vi "Save_full_Res_rows.vi"(2 "Selected Rows":i32[](array[numeric]), 3 "Filename to write":path, 4 "Filename Orig":path) -> ()   [LabVIEW 2020]
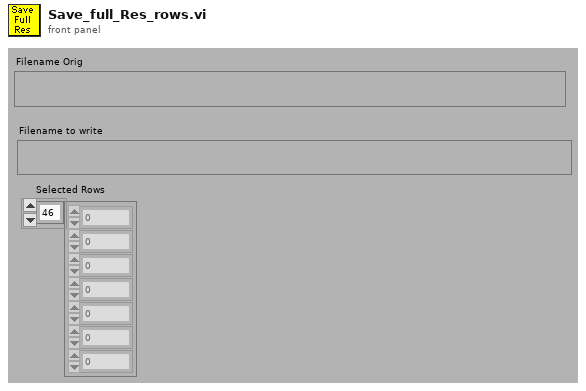
[diagram p1: front panel]
types:
  T1 = enum16{"read/write", "read-only", "write-only", "write-only (truncate)"}
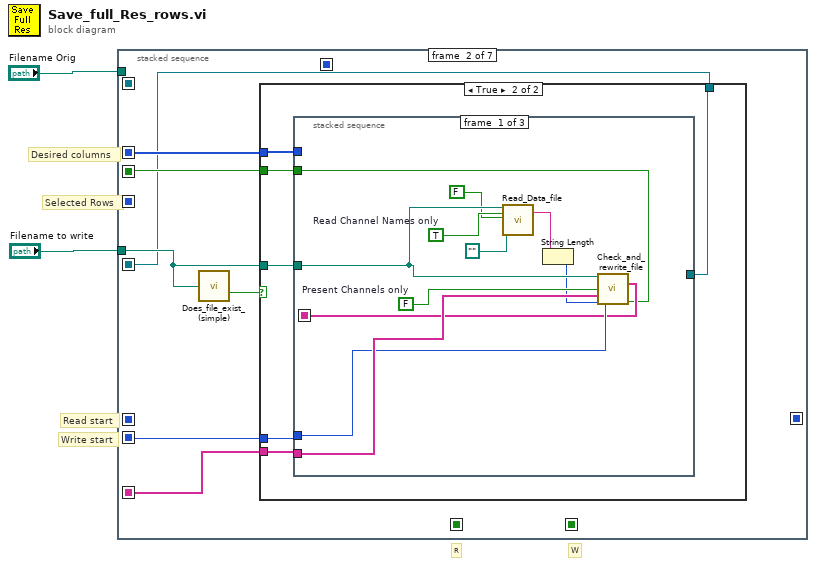
[diagram p0: block diagram]
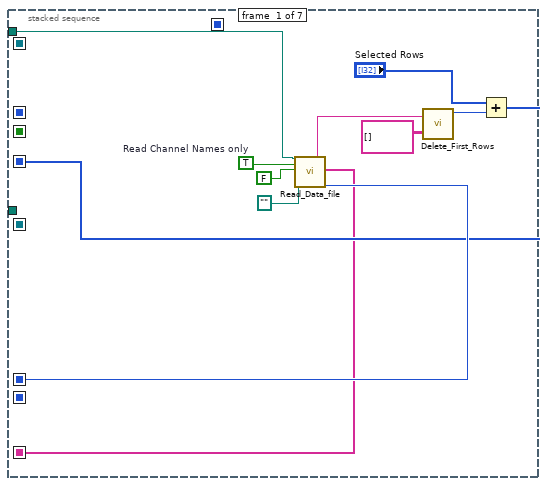
[diagram p2: hidden frame]
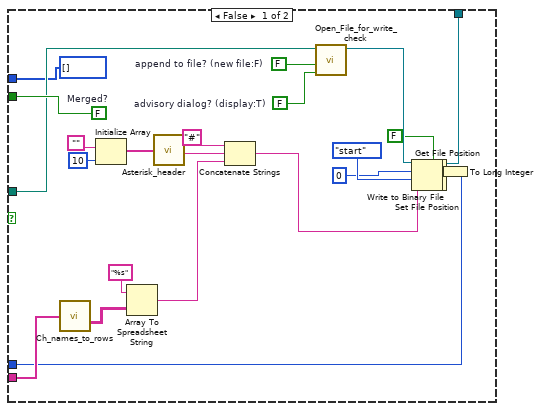
[diagram p3: hidden frame]
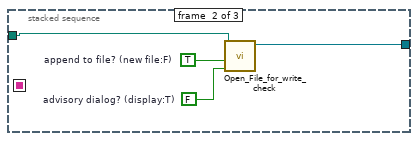
[diagram p4: hidden frame]
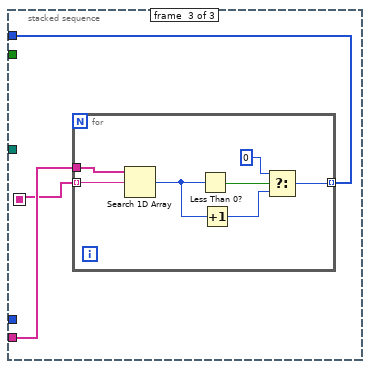
[diagram p5: hidden frame]
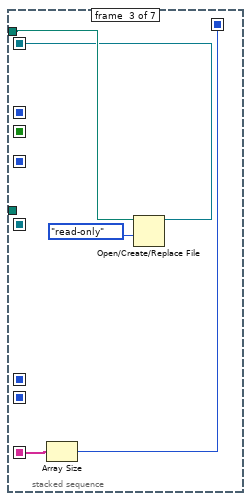
[diagram p6: hidden frame]
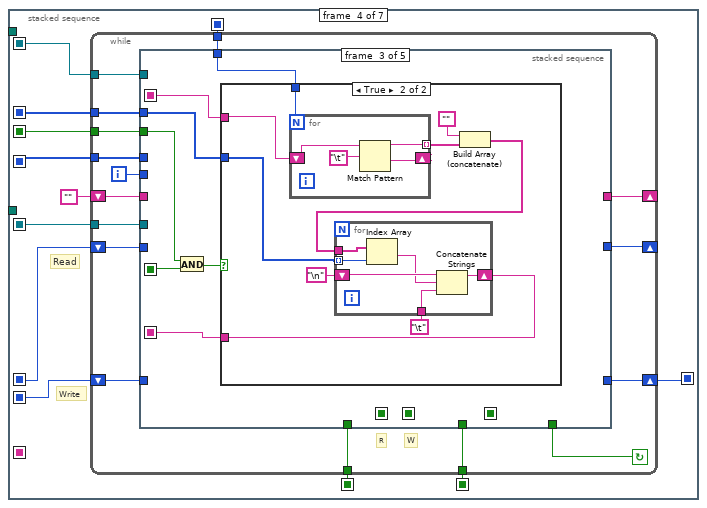
[diagram p7: hidden frame]
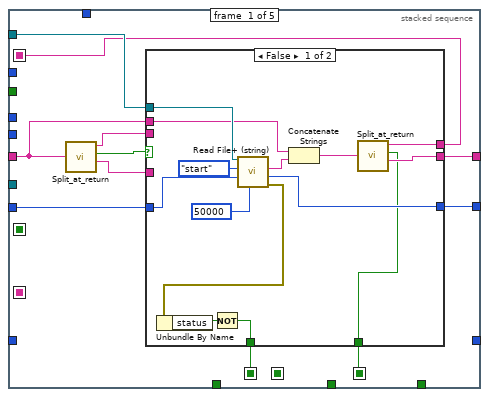
[diagram p8: hidden frame]
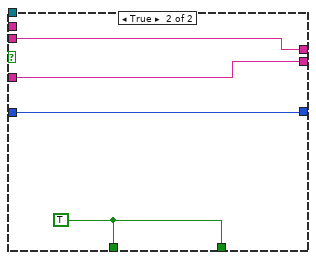
[diagram p9: hidden frame]
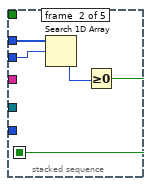
[diagram p10: hidden frame]
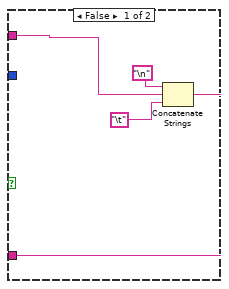
[diagram p11: hidden frame]
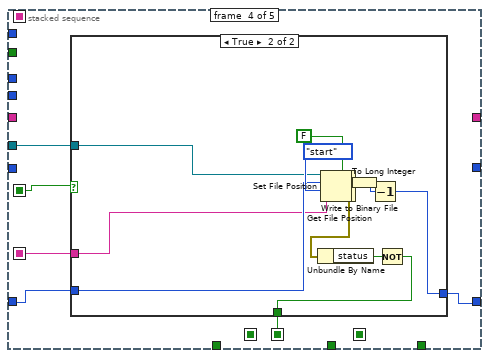
[diagram p12: hidden frame]
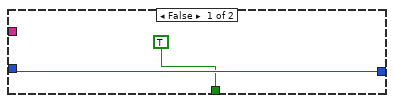
[diagram p13: hidden frame]
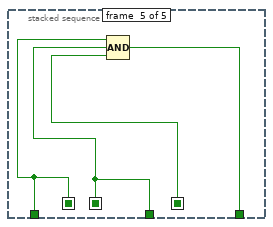
[diagram p14: hidden frame]
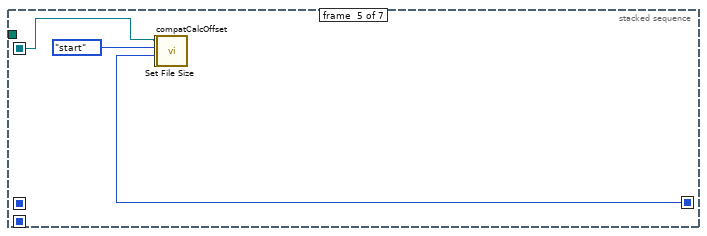
[diagram p15: hidden frame]
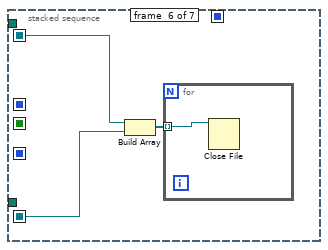
[diagram p16: hidden frame]
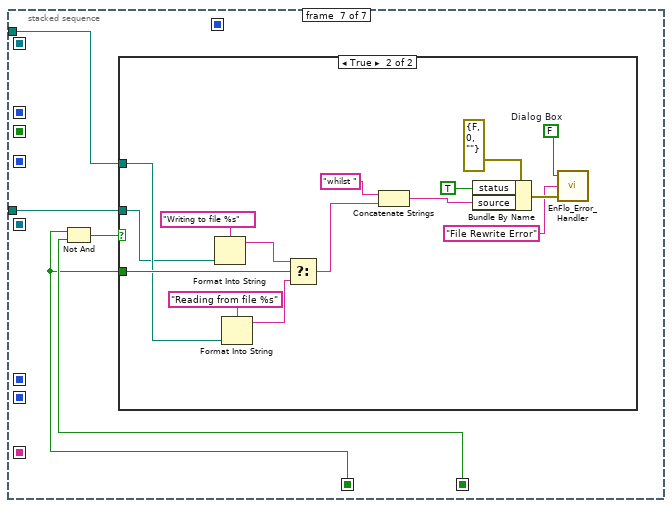
[diagram p17: hidden frame]
diagram:
  # "Desired columns"
  # "Selected Rows"
  # "Read start"
  # "Write start"
  # "W"
  # "R"
  n1 = stacked-sequence {
    seq-local: [_ _ w80 _ _ _ _] -> [_ _ _ w86 _ w209 _]
    seq-local: [w10 _ _ _ _ _ _] -> [_ _ _ w89 _ _ _]
    seq-local: [_ _ _ w93 _ _ _] -> [_ _ _ _ _ _ w213]
    seq-local: [_ _ _ w92 _ _ _] -> [_ _ _ _ _ _ w215]
    seq-local: [_ _ _ w91 _ _ _] -> [_ _ _ _ w206 _ _]
    seq-local: [w5 _ _ _ _ _ _] -> [_ _ _ w90 _ _ _]
    seq-local: [_ w16 _ _ _ _ _] -> [_ _ _ w88 _ _ _]
    seq-local: [w4 _ _ _ _ _ _] -> [_ w19 w79 _ _ _ _]
    seq-local: [_ w18 _ _ _ _ _] -> [_ _ _ w83 _ _ _]
    seq-local: [_ w17 _ _ _ _ _] -> [_ _ _ w84 _ _ _]
    seq-local: [_ w14 _ _ _ _ _] -> [_ _ _ w87 w204 w207 _]
    seq-local: [_ _ w78 _ _ _ _] -> [_ _ _ w85 _ _ _]
    tunnel: "Filename Orig" -> [w11 _ w81 _ _ _ w212]
    tunnel: "Filename to write" -> [_ w15 _ _ _ _ w211]
    frame #0 {
      w12 = TRUE  # Read Channel Names only
      n2 = call "Read_Data_file.vi"("Results file"=w11, "Read Channel Names only"=w12, "Delete First Rows?"=FALSE, "Template File"=path "") -> ("Filetype"=w9:string, "Ch names Out"=w4:string[], "mark after read (chars.)"=w10:i32)  [unwired: 3 in, 10 out]
      n3 = call "Delete_First_Rows.vi"("File Type (Default: AutoTrim)"=w9, "Data In"=string[][] []) -> ("Rows removed"=w8:i32)  [unwired: 2 out]
      n4 = Add(x="Selected Rows", y=w8) -> (x+y=w5:i32[])
    }
    frame #1 {
      n5 = call "Does_file_exist_(simple).vi"("Pathname"=w15) -> ("exists?"=w20:bool)
      n6 = case shown="True" w20 {
        tunnel: w15 -> [w34 w52]
        tunnel: w19 -> [w45 w51]
        tunnel: [i32[] [] w48] -> w18
        tunnel: [w46 w47] -> w17
        tunnel: [w28 w50] -> w16
        tunnel: [w29 w49] -> w14
        frame False {
          w35 = FALSE  # advisory dialog? (display:T)
          w36 = FALSE  # append to file? (new file:F)
          w46 = FALSE  # Merged?
          n7 = call "Ch_names_to_rows.vi"("Channel Names"=w45) -> ("3 Row names"=w38:string[][])
          n8 = Initialize Array("", 10 ("Dimension Size")) -> (w42:string[])
          n9 = Array To Spreadsheet String(array=w38, 3:"%s" ("format string")) -> (spreadsheet string=w37:string)  [unwired: 1 out]
          n10 = call "Asterisk_header.vi"("Channel names"=w42) -> ("Header string"=w41:string)
          n11 = Concatenate Strings("#" ("Substring"), w41, w37) -> (w30:string)
          n12 = call "Open_File_for_write_check.vi"("advisory dialog? (display:T)"=w35, "append to file? (new file:F)"=w36, "file path"=w34) -> ("refnum"=w31:refnum<file>)  [unwired: 8 out]
          n13 = Set File Position(offset (in bytes) (0)=0 ("pos offset (0)"), refnum=w31, from (0:start)=enum16{"start", "end", "current"}."start" ("pos mode (0:2)")) -> (refnum out=w26:refnum<file>, error out=w25:errorcluster)  [unwired: 1 in]
          n14 = Write to Binary File(file (use dialog)=w26, data=w30, error in=w25, 5:FALSE ("prepend array or string size? (T)")) -> (refnum out=w24:refnum<file>, error out=w23:errorcluster)  [unwired: 3 out]
          n15 = Get File Position(4:w23, 7:w24) -> (2:w22:i64, 3:w29:refnum<file>)  [unwired: 1 out]
          n16 = To Long Integer(number=w22) -> (32bit integer=w28:i32)
        }
        frame True {
          n17 = stacked-sequence {
            seq-local: [w60 _ _] -> [_ _ w69]
            tunnel: w52 -> [w56 w65 _]
            tunnel: w51 -> [w62 _ w70]
            tunnel: [w61 _ _] -> w50
            tunnel: [_ w64 _] -> w49
            tunnel: [_ _ w68] -> w48
            tunnel: [w59 _ _] -> w47
            frame #0 {
              w58 = TRUE  # Read Channel Names only
              w63 = FALSE  # Present Channels only
              n18 = call "Read_Data_file.vi"("Results file"=w56, "Read Channel Names only"=w58, "Delete First Rows?"=FALSE, "Template File"=path "") -> ("String Before"=w55:string)  [unwired: 3 in, 12 out]
              n19 = String Length(string=w55) -> (length=w54:i32)
              n20 = call "Check_and_rewrite_file.vi"("Filename"=w56, "Present Channels only"=w63, "Present Channels"=w62, "Start of read offset (chars.: 0)"=w54) -> ("Merged Channels"=w60:string[], "Current file size (bytes)"=w61:i64, "Merged?"=w59:bool)  [unwired: 9 out]
            }
            frame #1 {
              w66 = FALSE  # advisory dialog? (display:T)
              w67 = TRUE  # append to file? (new file:F)
              n21 = call "Open_File_for_write_check.vi"("advisory dialog? (display:T)"=w66, "append to file? (new file:F)"=w67, "file path"=w65) -> ("refnum"=w64:refnum<file>)  [unwired: 8 out]
            }
            frame #2 {
              n22 = for {
                tunnel: w70 -> [w77]
                tunnel: w69 -> [w76] mode=indexing
                tunnel: [w71] -> w68 mode=indexing
                n23 = Search 1D Array(1D array=w77, element=w76) -> (index of element=w74:i32)  [unwired: 1 out]
                n24 = Less Than 0?(x=w74) -> (x < 0?=w75:bool)
                n25 = Increment(x=w74) -> (x+1=w73:i32)
                n26 = Select(t=0, s=w75, f=w73) -> (s? t:f=w71:i32)
              }
            }
          }
        }
      }
    }
    frame #2 {
      n27 = Array Size(array=w79) -> (size(s)=w78:i32)
      n28 = Open/Create/Replace File(file path (use dialog)=w81, access (0:read/write)=T1."read-only" ("open mode (0)")) -> (refnum out=w80:refnum<file>)  [unwired: 1 in, 5 out]
    }
    frame #3 {
      # "Write"
      # "Read"
      n29 = while {
        tunnel: [w101] -> w92
        tunnel: [w102] -> w93
        shift-left: w88 -> [w105]
        shift-right: [w104] -> w91
        tunnel: w86 -> [w107]
        shift-left: w89 -> [w109]
        shift-right: [w108] -> _
        shift-left: "" -> [w110]
        shift-right: [w106] -> _
        tunnel: w90 -> [w100]
        tunnel: w87 -> [w98]
        tunnel: w85 -> [w97]
        tunnel: w84 -> [w96]
        tunnel: w83 -> [w95]
        i -> [w99]
        stop <- w103 continue-if-true
        # "R"
        # "W"
        n30 = stacked-sequence {
          seq-local: [w113 _ _ _ _] -> [_ _ w144 _ _]
          seq-local: [_ _ _ w176 _] -> [_ _ _ _ w197]
          seq-local: [w114 _ _ _ _] -> [_ _ _ _ w199]
          seq-local: [w115 _ _ _ _] -> [_ _ _ _ w198]
          seq-local: [_ w140 _ _ _] -> [_ _ w148 w179 _]
          seq-local: [_ _ w149 _ _] -> [_ _ _ w175 _]
          tunnel: w110 -> [w118 _ _ _ _]
          tunnel: w109 -> [w121 _ _ _ _]
          tunnel: [w120 _ _ _ _] -> w108
          tunnel: w107 -> [w119 _ _ _ _]
          tunnel: [w117 _ _ _ _] -> w106
          tunnel: w105 -> [_ _ _ w178 _]
          tunnel: [_ _ _ w177 _] -> w104
          tunnel: [_ _ _ _ w200] -> w103
          tunnel: [_ _ _ _ w198] -> w102
          tunnel: [_ _ _ _ w197] -> w101
          tunnel: w100 -> [_ w143 _ _ _]
          tunnel: w99 -> [_ w142 _ _ _]
          tunnel: w98 -> [_ _ _ w174 _]
          tunnel: w97 -> [_ _ w150 _ _]
          tunnel: w96 -> [_ _ w147 _ _]
          tunnel: w95 -> [_ _ w145 _ _]
          frame #0 {
            n31 = call "Split_at_return.vi"("String"=w118) -> ("before substring"=w112:string, "Matched?"=w111:bool, "after substring"=w116:string)  [unwired: 1 in, 1 out]
            n32 = case shown="False" w111 {
              tunnel: w121 -> [w135 w139]
              tunnel: [w133 w139] -> w120
              tunnel: w119 -> [w132 _]
              tunnel: w118 -> [w130 _]
              tunnel: [w128 w138] -> w117
              tunnel: w116 -> [_ w138]
              tunnel: [w125 w137] -> w115
              tunnel: [w123 w137] -> w114
              tunnel: [w124 w136] -> w113
              tunnel: w112 -> [_ w136]
              frame False {
                n33 = call <vilib>:"Read File+ (string).vi"("count"=50000, "pos offset (bytes:0)"=w135, "pos mode (rel. to current:2)"=enum16{"start", "end", "current"}."start", "refnum"=w132) -> ("error out"=w127:errorcluster, "mark after read (bytes)"=w133:i32, "string"=w131:string)  [unwired: 1 in, 4 out]
                n34 = Unbundle By Name(w127) -> ("status"=w126:bool)
                n35 = Not(x=w126) -> (.not. x?=w125:bool)
                n36 = Concatenate Strings(w130, w131) -> (w129:string)
                n37 = call "Split_at_return.vi"("String"=w129) -> ("before substring"=w124:string, "Matched?"=w123:bool, "after substring"=w128:string)  [unwired: 1 in, 1 out]
              }
              frame True {
                w137 = TRUE
              }
            }
          }
          frame #1 {
            n38 = Search 1D Array(1D array=w143, element=w142) -> (index of element=w141:i32)  [unwired: 1 out]
            n39 = Greater Or Equal To 0?(x=w141) -> (x >= 0?=w140:bool)
          }
          frame #2 {
            n40 = And(x=w147, y=w148) -> (x .and. y?=w146:bool)
            n41 = case shown="True" w146 {
              tunnel: w144 -> [w153 w158]
              tunnel: w145 -> [_ w157]
              tunnel: w150 -> [_ w156]
              tunnel: [w152 w155] -> w149
              frame False {
                n42 = Concatenate Strings("\n", w153, "\t") -> (w152:string)
              }
              frame True {
                n43 = for {
                  N: w156 -> [_]
                  shift-right: [w165] -> _
                  shift-left: w158 -> [w166]
                  tunnel: [w164] -> w159 mode=indexing
                  n44 = Match Pattern(string=w166, regular expression="\t") -> (before substring=w164:string, after substring=w165:string)  [unwired: 3 out]
                }
                n45 = Build Array (concatenate)("", w159) -> (w163:string[])
                n46 = for {
                  tunnel: w157 -> [w173] mode=indexing
                  tunnel: w163 -> [w172]
                  shift-right: [w168] -> w155
                  shift-left: "\n" -> [w171]
                  tunnel: "\t" -> [w169]
                  n47 = Index Array(array=w172, index=w173) -> (element=w170:string)
                  n48 = Concatenate Strings(w171, w170, w169) -> (w168:string)
                }
              }
            }
          }
          frame #3 {
            n49 = case shown="True" w179 {
              tunnel: w178 -> [w181 w194]
              tunnel: [w181 w193] -> w177
              tunnel: [TRUE w190] -> w176
              tunnel: w175 -> [_ w189]
              tunnel: w174 -> [_ w188]
              frame False {
              }
              frame True {
                n50 = Set File Position(offset (in bytes) (0)=w194, refnum=w188, from (0:start)=enum16{"start", "end", "current"}."start" ("pos mode (0:2)")) -> (refnum out=w187:refnum<file>, error out=w186:errorcluster)  [unwired: 1 in]
                n51 = Write to Binary File(file (use dialog)=w187, data=w189, error in=w186, 5:FALSE ("prepend array or string size? (T)")) -> (refnum out=w185:refnum<file>, error out=w184:errorcluster)  [unwired: 3 out]
                n52 = Get File Position(4:w184, 7:w185) -> (0:w191:errorcluster, 2:w183:i64)  [unwired: 1 out]
                n53 = Unbundle By Name(w191) -> ("status"=w192:bool)
                n54 = To Long Integer(number=w183) -> (32bit integer=w196:i32)
                n55 = Decrement(x=w196) -> (x-1=w193:i32)
                n56 = Not(x=w192) -> (.not. x?=w190:bool)
              }
            }
          }
          frame #4 {
            n57 = Compound Arithmetic op=AND(w198, w197, w199) -> (w200:bool)
          }
        }
      }
    }
    frame #4 {
      n58 = call <vilib>:"compatCalcOffset.vi"("pos offset (0)"=w206, "pos mode (0:1)"=enum16{"start", "end", "current"}."start", "refnum"=w204) -> ("error out"=w203:errorcluster, "offset"=w202:i32, "dup refnum"=w201:refnum<file>)  [unwired: 1 in, 5 out]
      n59 = Set File Size(4:w203, 6:w202, 7:w201) -> ()  [unwired: 2 out]
    }
    frame #5 {
      n60 = Build Array(w209, w207) -> (w208:refnum<file>[])
      n61 = for {
        tunnel: w208 -> [w210] mode=indexing
        n62 = Close File(refnum=w210) -> ()  [unwired: 1 in, 2 out]
      }
    }
    frame #6 {
      n63 = Not And(1:w215, 2:w213) -> (0:w214:bool)
      n64 = case shown="True" w214 {
        tunnel: w213 -> [_ w230]
        tunnel: w212 -> [_ w220]
        tunnel: w211 -> [_ w217]
        frame False {
        }
        frame True {
          w225 = FALSE  # Dialog Box
          n65 = Format Into String(format string="Writing to file %s", w217) -> (resulting string=w216:string)  [unwired: 2 in, 1 out]
          n66 = Format Into String(format string="Reading from file %s", w220) -> (resulting string=w219:string)  [unwired: 2 in, 1 out]
          n67 = Select(t=w216, s=w230, f=w219) -> (s? t:f=w228:string)
          n68 = Concatenate Strings("whilst ", w228) -> (w223:string)
          n69 = Bundle By Name(cluster=errorcluster {"status"=FALSE, "code"=0, "source"=""} ("error in (no error)"), "status"=TRUE ("Bundle Element"), "source"=w223) -> (w226:errorcluster)
          n70 = call "EnFlo_Error_Handler.vi"("error in (no error)"=w226, "Error Type"="File Rewrite Error", "Dialog Box (F)"=w225) -> ()  [unwired: 3 out]
        }
      }
    }
  }
